vi "zadanie_5.vi"() -> ()   [LabVIEW 2023]
panel:
  in  "stop":bool
  in  "Amplituda Y":dbl(slide) scale=0.0..10.0
  in  "Amplituda X":dbl(slide) scale=0.0..10.0
  in  "Częstotliwość Y":dbl(slide) scale=0.0..10.0
  in  "Częstotliwość X":dbl(slide) scale=0.0..10.0
  in  "Faza Y":dbl(slide) scale=0.0..180.0
  in  "Faza X":dbl(slide) scale=0.0..180.0
  out "XY Graph":cluster{"Y":dbl[], "Y":dbl[]}[](graph)
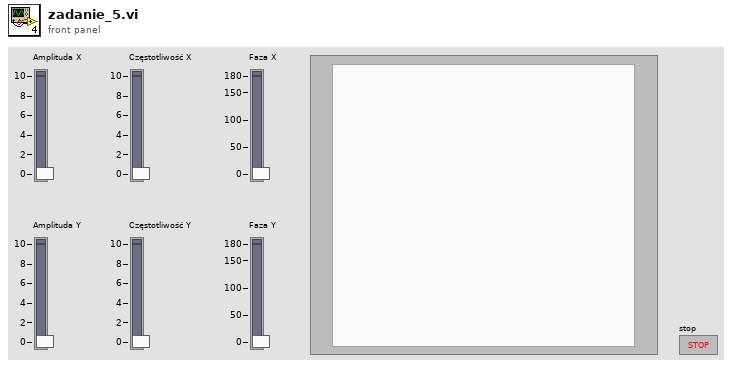
[diagram p1: front panel]
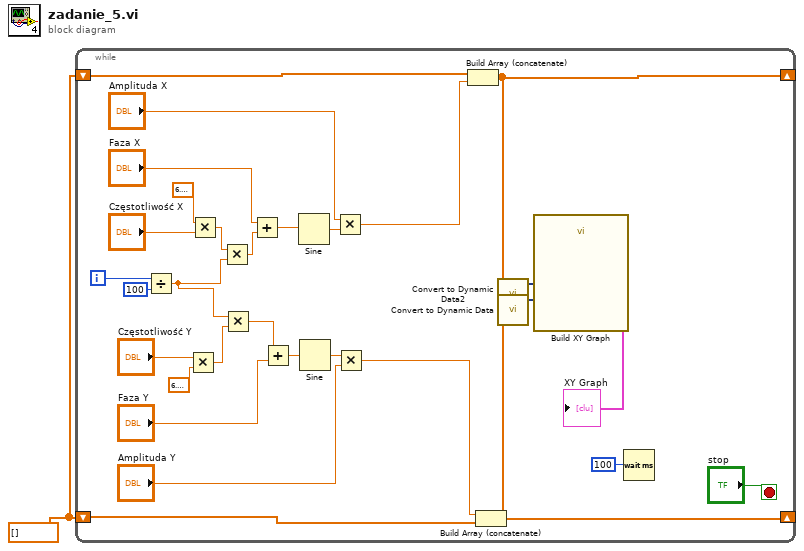
[diagram p0: block diagram]
diagram:
  w1 = dbl[] []
  n1 = while {
    shift-right: [w5] -> _
    shift-left: w1 -> [w10]
    shift-right: [w7] -> _
    shift-left: w1 -> [w8]
    i -> [w27]
    stop <- "stop" stop-if-true
    n2 = Divide(x=w27, y=100) -> (x/y=w23:dbl)
    n3 = Multiply(x="Częstotliwość Y", y=6.283185307179586) -> (x*y=w24:dbl)
    n4 = Multiply(x=6.283185307179586, y="Częstotliwość X") -> (x*y=w22:dbl)
    n5 = Multiply(x=w22, y=w23) -> (x*y=w20:dbl)
    n6 = Multiply(x=w23, y=w24) -> (x*y=w17:dbl)
    n7 = Add(x="Faza X", y=w20) -> (x+y=w19:dbl)
    n8 = Add(x=w17, y="Faza Y") -> (x+y=w13:dbl)
    n9 = Sine(x=w19) -> (sin(x)=w18:dbl)
    n10 = Sine(x=w13) -> (sin(x)=w14:dbl)
    n11 = Multiply(x="Amplituda X", y=w18) -> (x*y=w11:dbl)
    n12 = Multiply(x=w14, y="Amplituda Y") -> (x*y=w9:dbl)
    n13 = Build Array (concatenate)(w10, w11) -> (w5:dbl[])
    n14 = Build Array (concatenate)(w9, w8) -> (w7:dbl[])
    n15 = call "Convert to Dynamic Data2"("Array"=w5) -> ("Dynamic Data Type"=w4:dynamicdata)  [unwired: 3 in]
    n16 = call "Convert to Dynamic Data"("Array"=w7) -> ("Dynamic Data Type"=w6:dynamicdata)  [unwired: 3 in]
    n17 = call "Build XY Graph"("Y Input"=w6, "X Input"=w4) -> ("XY Graph"=→"XY Graph":cluster{"X":dbl[], "Y":dbl[]}[])  [unwired: 8 in, 1 out]
    n18 = Wait (ms)(milliseconds to wait=100) -> ()  [unwired: 1 out]
  }
